vi "SingleMeasurement.vi"(8 "error in (no error)":errorcluster, 11 "VISA resource name":refnum<visa-resource-name>) -> (0 "error out":errorcluster, 2 "output":dbl, 3 "VISA resource name out":refnum<visa-resource-name>)   [LabVIEW 2014, in "GP22_TDC_Arduinoed.lvlib"]
doc: "Take a single TDC measurement"
uses:
  GP22_TDC_Arduinoed.lvlib
  Private/ConvertTimes - Single.vi
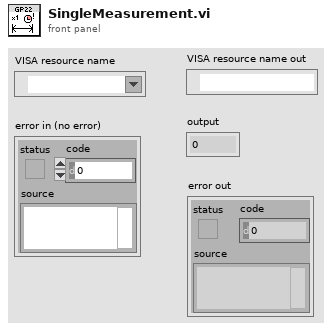
[diagram p1: front panel]
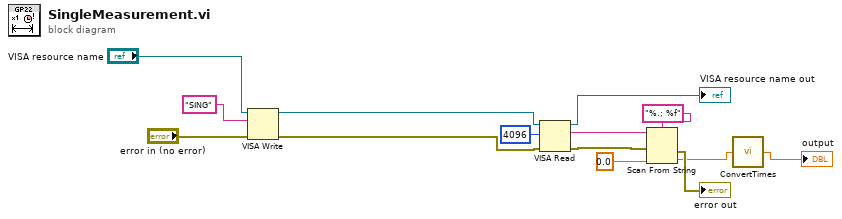
[diagram p0: block diagram]
diagram:
  n1 = VISA Write(VISA resource name="VISA resource name", write buffer="SING" ("command"), error in (no error)="error in (no error)") -> (VISA resource name out=w3:refnum<visa-resource-name>, error out=w12:errorcluster)  [unwired: 1 out]
  n2 = VISA Read(VISA resource name=w3, byte count=u32 4096, error in (no error)=w12) -> (VISA resource name out=→"VISA resource name out":refnum<visa-resource-name>, read buffer=w8:string, error out=w6:errorcluster)  [unwired: 1 out]
  n3 = Scan From String(format string="%.; %f", input string=w8, error in=w6, default 1=0.0 ("default value 1")) -> (error out=→"error out":errorcluster, output 1=w2:dbl)  [unwired: 1 in, 2 out]
  n4 = call-poly "ConvertTimes.vi"("GP22 Output"=w2) -> ("Time/s"=→"output":dbl)
